vi "SetValue.vi"(8 "error in":errorcluster, 10 "Value":string, 11 "Guid in":refnum<class "Guid.lvclass">) -> (0 "error out":errorcluster, 3 "Guid out":refnum<class "Guid.lvclass">)   [LabVIEW 2021, in "ProligentXMLGenerator.lvlib" / "Guid.lvclass"]
uses:
  Guid.lvclass
  Guid.lvclass/Guid.ctl
  <vilib>/regexp/Match Regular Expression.xnode
  NonEmptyString/NonEmptyString.lvclass
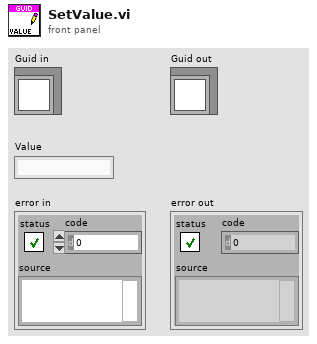
[diagram p1: front panel]
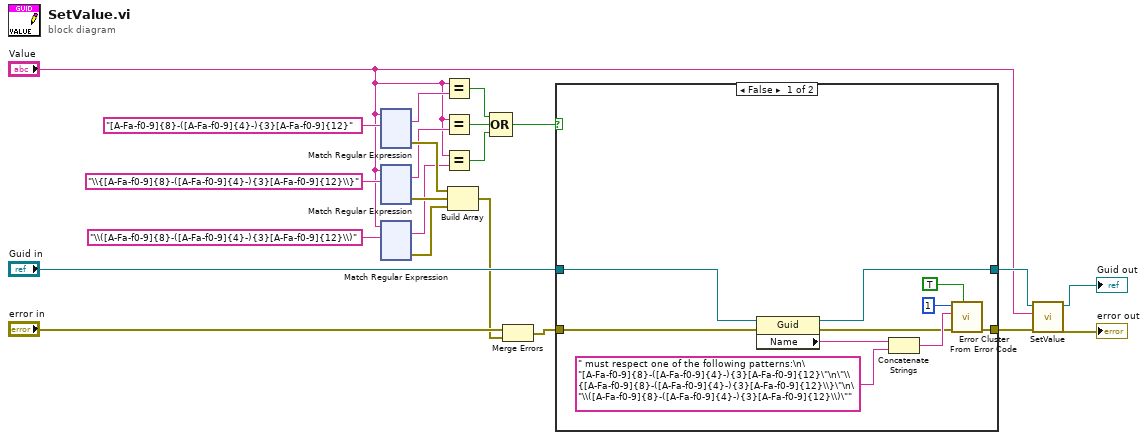
[diagram p0: block diagram]
diagram:
  n1 = xnode "Match Regular Expression"("input string"="Value", "regular expression"="[A-Fa-f0-9]{8}-([A-Fa-f0-9]{4}-){3}[A-Fa-f0-9]{12}" ("string")) -> ("whole match"=w8:string, "error out"=w13:errorcluster)  [unwired: 4 in, 3 out]
  n2 = xnode "Match Regular Expression"("input string"="Value", "regular expression"="\\{[A-Fa-f0-9]{8}-([A-Fa-f0-9]{4}-){3}[A-Fa-f0-9]{12}\\}" ("string")) -> ("whole match"=w9:string, "error out"=w12:errorcluster)  [unwired: 4 in, 3 out]
  n3 = xnode "Match Regular Expression"("input string"="Value", "regular expression"="\\([A-Fa-f0-9]{8}-([A-Fa-f0-9]{4}-){3}[A-Fa-f0-9]{12}\\)" ("string")) -> ("whole match"=w10:string, "error out"=w11:errorcluster)  [unwired: 4 in, 3 out]
  n4 = Equal?(x="Value", y=w8) -> (x = y?=w7:bool)
  n5 = Equal?(x="Value", y=w9) -> (x = y?=w6:bool)
  n6 = Equal?(x="Value", y=w10) -> (x = y?=w5:bool)
  n7 = Build Array(w13, w12, w11) -> (w1:errorcluster[])
  n8 = Compound Arithmetic op=OR(w7, w6, w5) -> (w4:bool)
  n9 = Merge Errors("error in", w1) -> (w2:errorcluster)
  n10 = case shown="False" w4 {
    tunnel: "Guid in" -> [w29 w34]
    tunnel: [w25 w34] -> w17
    tunnel: w2 -> [w31 w33]
    tunnel: [w30 w33] -> w20
    frame False {
      n11 = property on="Property Node" class="Guid"(reference=w29, error in=w31) -> (reference out=w25:refnum<class "Guid.lvclass">, error out=w23:errorcluster, "Name"=w28:string)
      n12 = Concatenate Strings(w28, " must respect one of the following patterns:\n\"[A-Fa-f0-9]{8}-([A-Fa-f0-9]{4}-){3}[A-Fa-f0-9]{12}\"\n\"\\{[A-Fa-f0-9]{8}-([A-Fa-f0-9]{4}-){3}[A-Fa-f0-9]{12}\\}\"\n\"\\([A-Fa-f0-9]{8}-([A-Fa-f0-9]{4}-){3}[A-Fa-f0-9]{12}\\)\"" ("string")) -> (w27:string)
      n13 = call <vilib>:"Error Cluster From Error Code.vi"("show call chain? (False)"=TRUE, "error in (no error)"=w23, "error message (\"\")"=w27, "error code (0)"=1) -> ("error out"=w30:errorcluster)  [unwired: 5 in]
    }
    frame True {
    }
  }
  n14 = call-parent "SetValue.vi"("error in"=w20, "Value"="Value", "NonEmptyString in"=w17) -> ("error out"=→"error out":errorcluster, "NonEmptyString out"=→"Guid out":refnum<class "Guid.lvclass">)  [unwired: 7 in]
